vi "svc_Clear Error Cluster for Specific Code.vi"(11 "error in (no error)":errorcluster, 12 "code":i32=1984) -> (14 "error cleared":bool, 15 "error out":errorcluster)   [LabVIEW 2017]
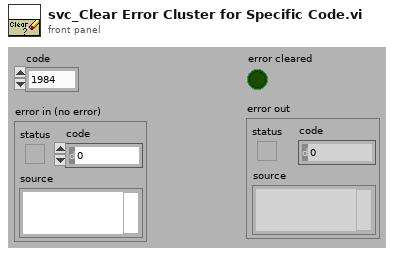
[diagram p1: front panel]
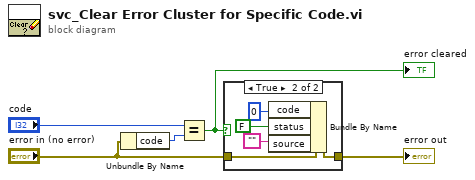
[diagram p0: block diagram]
diagram:
  n1 = Unbundle By Name("error in (no error)") -> ("code"=w2:i32)
  n2 = Equal?(x="code", y=w2) -> (x = y?=w1:bool)
  "error cleared" <- w1
  n3 = case shown="True" w1 {
    tunnel: "error in (no error)" -> [w6 w11]
    tunnel: [w6 w10] -> w4
    frame False {
    }
    frame True {
      n4 = Bundle By Name(cluster=w11, "code"=0, "status"=FALSE, "source"="") -> (w10:errorcluster)
    }
  }
  "error out" <- w4
